vi "Generate Unique Header.vi"(8 "error in":errorcluster, 11 "xData in":refnum<class "xData.lvclass">) -> (0 "error out":errorcluster, 2 "Header":string[](array[string]), 3 "xData out":refnum<class "xData.lvclass">)   [LabVIEW 2014, in "xData.lvclass"]
uses:
  xData.lvclass
  reusable/Data/Data.lvclass
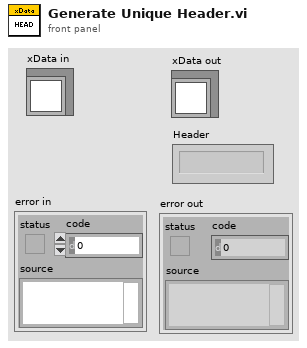
[diagram p1: front panel]
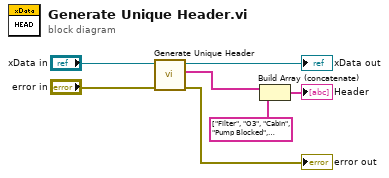
[diagram p0: block diagram]
diagram:
  n1 = call-parent "Generate Unique Header.vi"("error in"="error in", "Data in"="xData in") -> ("error out"=→"error out":errorcluster, "Header"=w4:string[], "Data out"=→"xData out":refnum<class "xData.lvclass">)  [unwired: 7 in]
  n2 = Build Array (concatenate)(w4, string[] ["Filter", "O3", "Cabin", "Pump Blocked", "Interlock", "Impactor Blocked"] ("array")) -> (→"Header":string[])
